vi "fgv_debug.vi"(7 "Operation":enum16{"Reset", "ReadCommand", "SetCommand"}(ring)=enum."ReadCommand", 8 "error in":errorcluster, 9 "Command in":string, 11 "VISA resource name":refnum<visa-resource-name>) -> (0 "error out":errorcluster, 3 "VISA resource name out":refnum<visa-resource-name>)   [LabVIEW 2014, in "rszvl_rsidr_core.lvlib"]
uses:
  rszvl_rsidr_core.lvlib
  type_Error_Codes.ctl
  Match Regular Expression.xnode
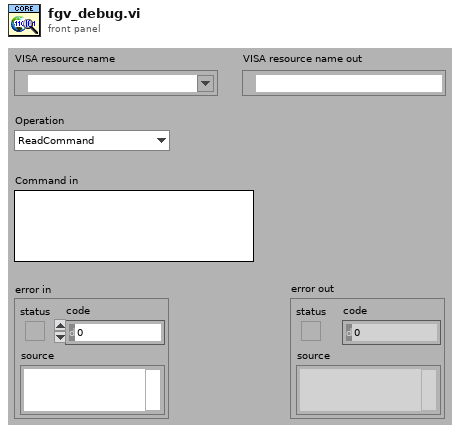
[diagram p1: front panel]
types:
  T1 = typedef "rszvl_rsidr_core.lvlib/type_Error_Codes.ctl" = enum16{"No_error", "VISA_err_ResourceNotFound", "VISA_err_Timeout", "VISA_warn_MoreDataAvailable", "RS_err_MissingCallback", "RS_err_InvalidAttribute", "RS_err_InvalidValue", "RS_err_UnknownResource", "RS_err_AlreadyInitialized", "RS_err_InstrumentStatus", "RS_err_BadRepCapName", "RS_err_TypesMismatch", "RS_err_ValueNotSupported", "RS_err_InvalidRngTable", "RS_err_IDqueryFail", "RS_err_UnexpResponse", "VISA_warn_ConfigNotLoaded", "RS_err_AttributeNotReadable", "RS_err_AttributeNotWritable", "RS_err_InstrumentType", "RS_err_InstrumentOption", "VISA_err_InvalidSize", "RS_err_ReliabilityIndicator", "VISA_warn_UnknownStatus", "VISA_warn_TermCharRead", "VISA_err_IO_error"}
  T2 = typedef "rszvl_rsidr_core.lvlib/type_Session_Data.ctl" = cluster{"Instr type":string, "Instr type for err. msg.":string, "Installed Options":string[], "OPC Timeout":i32, "Query Instrument Status":bool, "Check Range":bool, "Check Options":bool, "Add LF to Write":bool, "Simulate":bool, "Logging":bool, "Logging params":variant, "Interface Type":enum16{"Unknown", "GPIB", "VXI", "GPIB_VXI", "ASRL", "PXI", "TCPIP", "USB", "SOCKET"}, "Fast Sweep":i32, "AdditionalFlags":i32, "WaitBeforeWrite":i32, "WaitBeforeRead":i32, "BinDataChunkSize":i64}
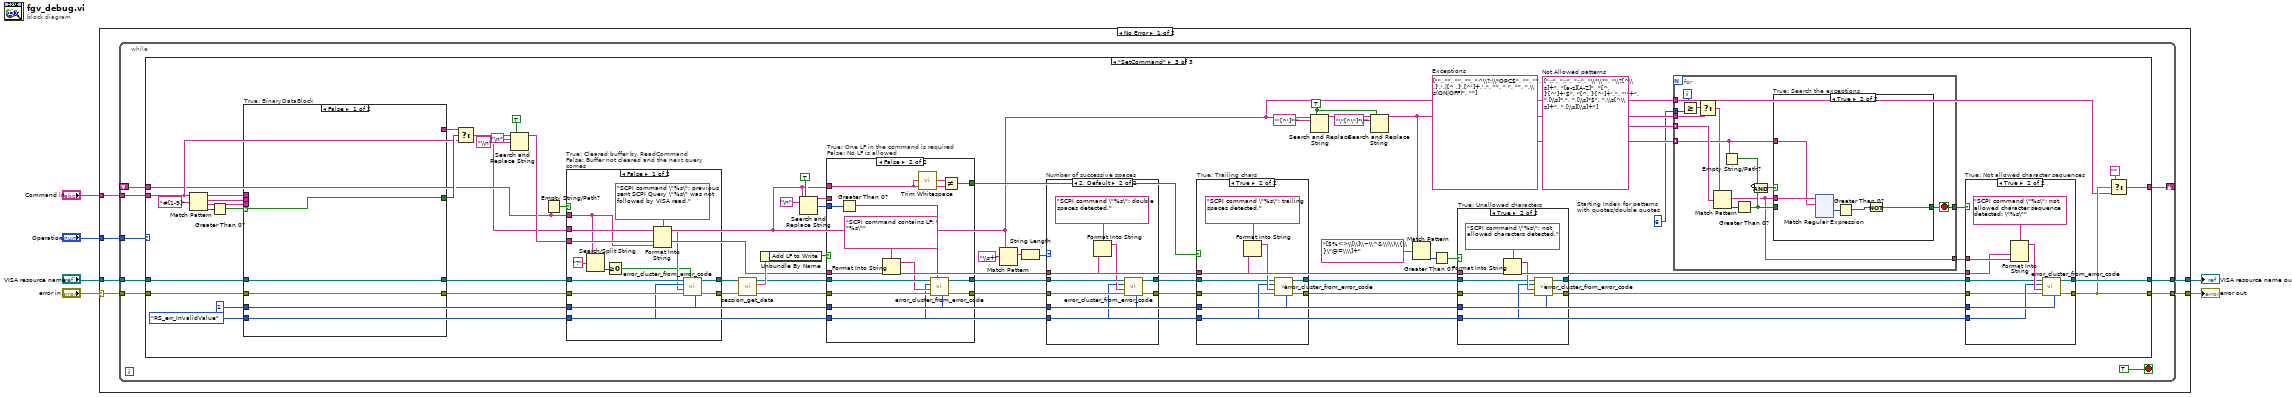
[diagram p0: block diagram]
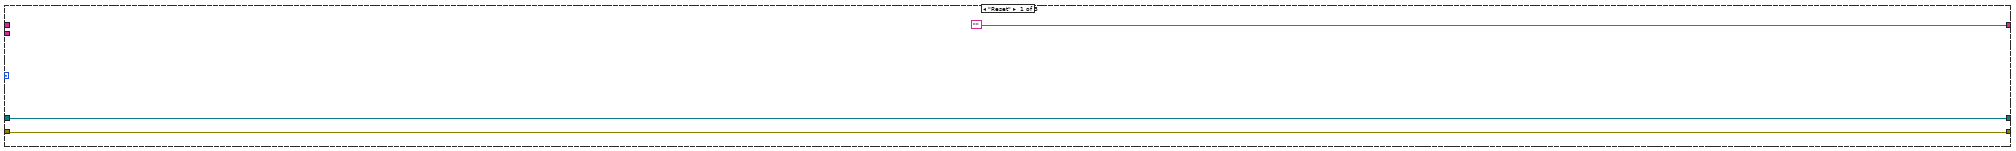
[diagram p2: hidden frame]
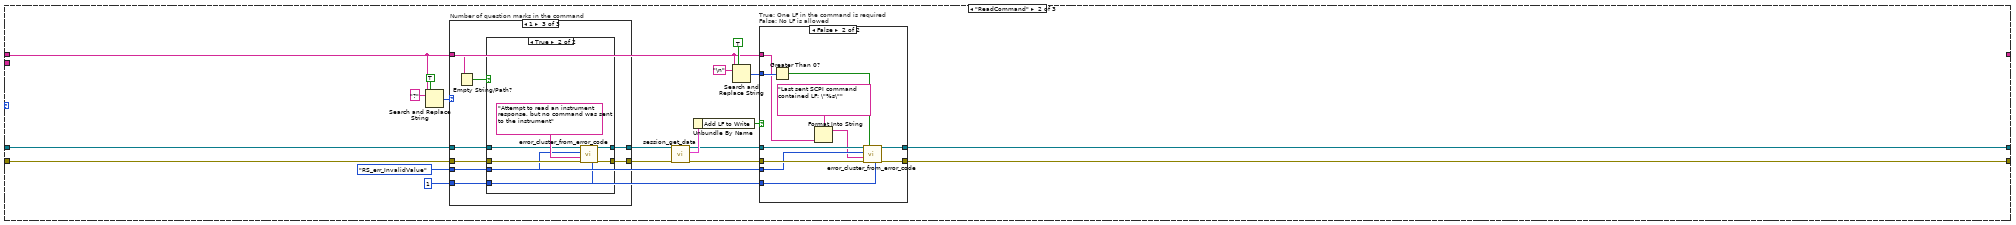
[diagram p3: hidden frame]
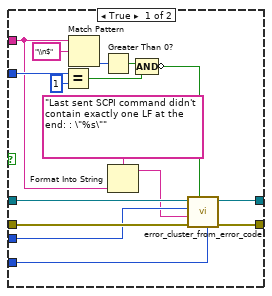
[diagram p4: hidden frame]
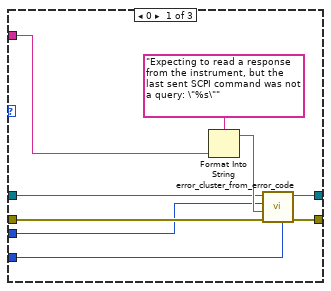
[diagram p5: hidden frame]
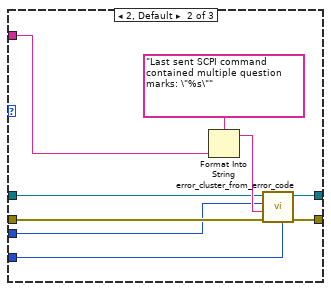
[diagram p6: hidden frame]
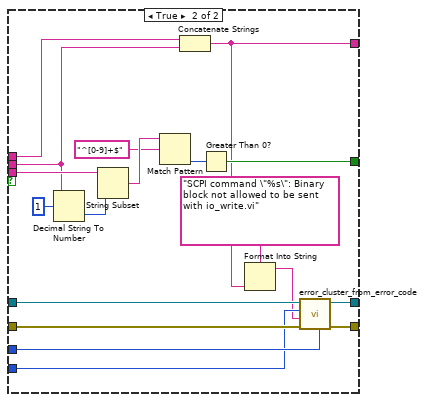
[diagram p8: hidden frame]
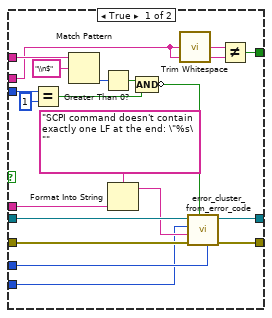
[diagram p13: hidden frame]
diagram:
  n1 = case shown="No Error" "error in" {
    selector: "error in" -> [w8 w414]
    tunnel: [w10 w414] -> w2
    tunnel: "Operation" -> [w12 _]
    tunnel: "Command in" -> [w11 _]
    tunnel: "VISA resource name" -> [w7 w413]
    tunnel: [w9 w413] -> w1
    frame No Error {
      n2 = while {
        shift-right: [w18] -> _
        shift-left: _ -> [w17]
        tunnel: w12 -> [w20]
        tunnel: w8 -> [w14]
        tunnel: w11 -> [w19]
        tunnel: w7 -> [w13]
        tunnel: [w16] -> w10
        tunnel: [w15] -> w9
        stop <- TRUE stop-if-true
        n3 = case shown="\"SetCommand\"" w20 {
          tunnel: w19 -> [_ _ w125]
          tunnel: ["" ("Empty String Constant") _ w161] -> w18
          tunnel: w17 -> [_ w28 w124]
          tunnel: w14 -> [w23 w40 w110]
          tunnel: w13 -> [w22 w39 w109]
          tunnel: [w23 w27 w140] -> w16
          tunnel: [w22 w26 w141] -> w15
          frame "Reset" {
          }
          frame "ReadCommand" {
            w25 = 1 ("Cut first x elements\nfrom Error Chain (0)")
            w31 = type_Error_Codes."RS_err_InvalidValue" ("Error Enum in")
            n4 = Search and Replace String(replace all?=TRUE ("replace all? (F)"), input string=w28, search string="?") -> (number of replacements=w41:i32)  [unwired: 5 in, 3 out]
            n5 = case "Number of question marks in the command" shown="1" w41 {
              tunnel: w40 -> [w78 w87 w94]
              tunnel: [w77 w86 w92] -> w38
              tunnel: w28 -> [w76 w85 w96]
              tunnel: w39 -> [w74 w82 w93]
              tunnel: [w73 w84 w91] -> w37
              tunnel: w31 -> [w72 w81 w90]
              tunnel: w25 -> [w71 w80 w89]
              frame 0 {
                n6 = Format Into String(format string="Expecting to read a response from the instrument, but the last sent SCPI command was not a query: \"%s\"", w76) -> (resulting string=w75:string)  [unwired: 2 in, 1 out]
                n7 = call "error_cluster_from_error_code.vi"("Cut first x elements\nfrom Error Chain (0)"=w71, "error in"=w78, "error message (\"\")"=w75, "Error Enum in"=w72, "VISA resource name"=w74) -> ("error out"=w77:errorcluster, "VISA resource name out"=w73:refnum<visa-resource-name>)  [unwired: 5 in]
              }
              frame 2, Default {
                n8 = Format Into String(format string="Last sent SCPI command contained multiple question marks: \"%s\"", w85) -> (resulting string=w83:string)  [unwired: 2 in, 1 out]
                n9 = call "error_cluster_from_error_code.vi"("Cut first x elements\nfrom Error Chain (0)"=w80, "error in"=w87, "error message (\"\")"=w83, "Error Enum in"=w81, "VISA resource name"=w82) -> ("error out"=w86:errorcluster, "VISA resource name out"=w84:refnum<visa-resource-name>)  [unwired: 5 in]
              }
              frame 1 {
                n10 = Empty String/Path?(string/path=w96) -> (empty?=w95:bool)
                n11 = case shown="True" w95 {
                  tunnel: w94 -> [w98 w104]
                  tunnel: [w98 w102] -> w92
                  tunnel: w93 -> [w97 w103]
                  tunnel: [w97 w101] -> w91
                  tunnel: w90 -> [_ w100]
                  tunnel: w89 -> [_ w99]
                  frame False {
                  }
                  frame True {
                    n12 = call "error_cluster_from_error_code.vi"("Cut first x elements\nfrom Error Chain (0)"=w99, "error in"=w104, "error message (\"\")"="Attempt to read an instrument response, but no command was sent to the instrument" ("error message (\"\")"), "Error Enum in"=w100, "VISA resource name"=w103) -> ("error out"=w102:errorcluster, "VISA resource name out"=w101:refnum<visa-resource-name>)  [unwired: 5 in]
                  }
                }
              }
            }
            n13 = call "session_get_data.vi"("error in"=w38, "VISA resource name"=w37) -> ("error out"=w33:errorcluster, "Session User Data out"=w34:T2, "VISA resource name out"=w32:refnum<visa-resource-name>)  [unwired: 7 in]
            n14 = Unbundle By Name(w34) -> ("Add LF to Write"=w30:bool)
            n15 = Search and Replace String(replace all?=TRUE ("replace all? (F)"), input string=w28, search string="\n" ("Line Feed Constant")) -> (number of replacements=w29:i32)  [unwired: 5 in, 3 out]
            n16 = case "True: One LF in the command is required\nFalse: No LF is allowed" shown="False" w30 {
              tunnel: w33 -> [w59 w70]
              tunnel: w32 -> [w58 w69]
              tunnel: w31 -> [w57 w68]
              tunnel: w29 -> [w56 w65]
              tunnel: w28 -> [w46 w61]
              tunnel: [w49 w67] -> w27
              tunnel: [w48 w66] -> w26
              tunnel: w25 -> [w44 w60]
              frame True {
                n17 = Equal?(x=w56, y=1) -> (x = y?=w51:bool)
                n18 = Match Pattern(string=w46, regular expression="\\n$") -> (offset past match=w53:i32)  [unwired: 1 in, 3 out]
                n19 = Greater Than 0?(x=w53) -> (x > 0?=w52:bool)
                n20 = Format Into String(format string="Last sent SCPI command didn't contain exactly one LF at the end: : \"%s\"", w46) -> (resulting string=w45:string)  [unwired: 2 in, 1 out]
                n21 = Compound Arithmetic op=AND(w52, w51) -> (invert w50:bool)
                n22 = call "error_cluster_from_error_code.vi"("Cut first x elements\nfrom Error Chain (0)"=w44, "error creation enabled (T)"=w50, "error in"=w59, "error message (\"\")"=w45, "Error Enum in"=w57, "VISA resource name"=w58) -> ("error out"=w49:errorcluster, "VISA resource name out"=w48:refnum<visa-resource-name>)  [unwired: 4 in]
              }
              frame False {
                n23 = Greater Than 0?(x=w65) -> (x > 0?=w64:bool)
                n24 = Format Into String(format string="Last sent SCPI command contained LF: \"%s\"", w61) -> (resulting string=w62:string)  [unwired: 2 in, 1 out]
                n25 = call "error_cluster_from_error_code.vi"("Cut first x elements\nfrom Error Chain (0)"=w60, "error creation enabled (T)"=w64, "error in"=w70, "error message (\"\")"=w62, "Error Enum in"=w68, "VISA resource name"=w69) -> ("error out"=w67:errorcluster, "VISA resource name out"=w66:refnum<visa-resource-name>)  [unwired: 4 in]
              }
            }
          }
          frame "SetCommand" {
            w116 = 6  # Starting Index for patterns with quotes/double quotes
            w130 = string[] ["", "", "", "", "^\\?;\\*OPC$", "", "", "[^ ,]','.|[^ ,]',[^']+,'.", "", " ", "", ",\\s(ON|OFF)", ""]  # Exceptions
            w121 = TRUE ("replace all? (F)")
            w145 = string[] ["::", ";;", ":;", "\\*\\*", "\\?[^\\s]+", "[a-z][A-Z]", "[^, ]'[^']+'$", "[^, ]'[^']+'.", "''+", ",[\\s]*,", ",[\\s]*$", ",\\s[^\\s]+", ",[\\s][\\s]+"]  # Not Allowed patterns
            w111 = 1 ("Cut first x elements\nfrom Error Chain (0)")
            w106 = type_Error_Codes."RS_err_InvalidValue" ("Error Enum in")
            n26 = Match Pattern(string=w125, regular expression="#[1-9]") -> (before substring=w113:string, match substring=w115:string, after substring=w127:string, offset past match=w129:i32)  [unwired: 1 in]
            n27 = Greater Than 0?(x=w129) -> (x > 0?=w128:bool)
            n28 = case "True: BinaryDataBlock" shown="False" w128 {
              selector: w128 -> [w169 _]
              tunnel: w127 -> [_ w186]
              tunnel: w115 -> [_ w179]
              tunnel: [w169 w181] -> w126
              tunnel: [_ w170] -> w114
              tunnel: w113 -> [_ w180]
              tunnel: w111 -> [_ w174]
              tunnel: w110 -> [w167 w178]
              tunnel: w109 -> [w168 w177]
              tunnel: [w167 w176] -> w108
              tunnel: [w168 w175] -> w107
              tunnel: w106 -> [_ w173]
              frame False {
              }
              frame True {
                n29 = Decimal String To Number(string=w179, offset=1) -> (number=w185:i32)  [unwired: 1 in, 1 out]
                n30 = String Subset(string=w186, length (rest)=w185) -> (substring=w184:string)  [unwired: 1 in]
                n31 = Match Pattern(string=w184, regular expression="^[0-9]+$") -> (offset past match=w182:i32)  [unwired: 1 in, 3 out]
                n32 = Concatenate Strings(w180, w179) -> (w170:string)
                n33 = Greater Than 0?(x=w182) -> (x > 0?=w181:bool)
                n34 = Format Into String(format string="SCPI command \"%s\": Binary block not allowed to be sent with io_write.vi", w170) -> (resulting string=w171:string)  [unwired: 2 in, 1 out]
                n35 = call "error_cluster_from_error_code.vi"("Cut first x elements\nfrom Error Chain (0)"=w174, "error in"=w178, "error message (\"\")"=w171, "Error Enum in"=w173, "VISA resource name"=w177) -> ("error out"=w176:errorcluster, "VISA resource name out"=w175:refnum<visa-resource-name>)  [unwired: 5 in]
              }
            }
            n36 = Select(t=w114, s=w126, f=w125) -> (s? t:f=w117:string)
            n37 = Search and Replace String(replace all?=TRUE ("replace all? (F)"), input string=w117, search string="\n" ("Line Feed Constant"), replace string="\\n" ("input string")) -> (result string=w132:string)  [unwired: 4 in, 3 out]
            n38 = Empty String/Path?(string/path=w124) -> (empty?=w162:bool)
            n39 = case "True: Cleared buffer by ReadCommand\nFalse: Buffer not cleared and the next query comes" shown="False" w162 {
              tunnel: w124 -> [w405 _]
              tunnel: w108 -> [w409 w412]
              tunnel: [w408 w412] -> w152
              tunnel: w117 -> [_ _]
              tunnel: w111 -> [w404 _]
              tunnel: w106 -> [w403 _]
              tunnel: w107 -> [w402 w411]
              tunnel: [w401 w411] -> w153
              tunnel: w132 -> [w398 _]
              frame False {
                n40 = Search/Split String(string=w405, search string/char (-)="?") -> (offset of match=w407:i32)  [unwired: 1 in, 2 out]
                n41 = Greater Or Equal To 0?(x=w407) -> (x >= 0?=w399:bool)
                n42 = Format Into String(format string="SCPI command \"%s\": previous sent SCPI Query \"%s\" was not followed by VISA read.", w398, w405) -> (resulting string=w400:string)  [unwired: 2 in, 1 out]
                n43 = call "error_cluster_from_error_code.vi"("Cut first x elements\nfrom Error Chain (0)"=w404, "error creation enabled (T)"=w399, "error in"=w409, "error message (\"\")"=w400, "Error Enum in"=w403, "VISA resource name"=w402) -> ("error out"=w408:errorcluster, "VISA resource name out"=w401:refnum<visa-resource-name>)  [unwired: 4 in]
              }
              frame True {
              }
            }
            n44 = call "session_get_data.vi"("error in"=w152, "VISA resource name"=w153) -> ("error out"=w157:errorcluster, "Session User Data out"=w158:T2, "VISA resource name out"=w156:refnum<visa-resource-name>)  [unwired: 7 in]
            n45 = Unbundle By Name(w158) -> ("Add LF to Write"=w155:bool)
            n46 = Search and Replace String(replace all?=TRUE ("replace all? (F)"), input string=w117, search string="\n" ("Line Feed Constant")) -> (result string=w119:string, number of replacements=w154:i32)  [unwired: 5 in, 2 out]
            n47 = case "True: One LF in the command is required\nFalse: No LF is allowed" shown="False" w155 {
              tunnel: w157 -> [w372 w386]
              tunnel: w156 -> [w371 w385]
              tunnel: w154 -> [w370 w382]
              tunnel: w117 -> [w360 w374]
              tunnel: [w363 w384] -> w150
              tunnel: [w362 w383] -> w151
              tunnel: w111 -> [w358 w378]
              tunnel: w106 -> [w357 w377]
              tunnel: w132 -> [w356 w376]
              tunnel: w119 -> [w354 _]
              tunnel: [w353 w373] -> w118
              frame True {
                n48 = Equal?(x=w370, y=1) -> (x = y?=w365:bool)
                n49 = Match Pattern(string=w360, regular expression="\\n$") -> (offset past match=w367:i32)  [unwired: 1 in, 3 out]
                n50 = Greater Than 0?(x=w367) -> (x > 0?=w366:bool)
                n51 = Format Into String(format string="SCPI command doesn't contain exactly one LF at the end: \"%s\"", w356) -> (resulting string=w359:string)  [unwired: 2 in, 1 out]
                n52 = Compound Arithmetic op=AND(w366, w365) -> (invert w364:bool)
                n53 = call "Trim Whitespace.vi"("string"=w354) -> ("trimmed string"=w355:string)  [unwired: 1 in]
                n54 = call "error_cluster_from_error_code.vi"("Cut first x elements\nfrom Error Chain (0)"=w358, "error creation enabled (T)"=w364, "error in"=w372, "error message (\"\")"=w359, "Error Enum in"=w357, "VISA resource name"=w371) -> ("error out"=w363:errorcluster, "VISA resource name out"=w362:refnum<visa-resource-name>)  [unwired: 4 in]
                n55 = Not Equal?(x=w355, y=w354) -> (x != y?=w353:bool)
              }
              frame False {
                n56 = Greater Than 0?(x=w382) -> (x > 0?=w381:bool)
                n57 = Format Into String(format string="SCPI command contains LF: \"%s\"", w376) -> (resulting string=w379:string)  [unwired: 2 in, 1 out]
                n58 = call "Trim Whitespace.vi"("string"=w374) -> ("trimmed string"=w375:string)  [unwired: 1 in]
                n59 = call "error_cluster_from_error_code.vi"("Cut first x elements\nfrom Error Chain (0)"=w378, "error creation enabled (T)"=w381, "error in"=w386, "error message (\"\")"=w379, "Error Enum in"=w377, "VISA resource name"=w385) -> ("error out"=w384:errorcluster, "VISA resource name out"=w383:refnum<visa-resource-name>)  [unwired: 4 in]
                n60 = Not Equal?(x=w375, y=w374) -> (x != y?=w373:bool)
              }
            }
            n61 = Match Pattern(string=w117, regular expression="\\s+") -> (match substring=w165:string)  [unwired: 1 in, 3 out]
            n62 = String Length(string=w165) -> (length=w166:i32)
            n63 = case "Number of successive spaces" shown="2, Default" w166 {
              tunnel: w150 -> [w388 w397]
              tunnel: [w388 w396] -> w139
              tunnel: w151 -> [w387 w394]
              tunnel: [w387 w393] -> w138
              tunnel: w111 -> [_ w391]
              tunnel: w106 -> [_ w390]
              tunnel: w132 -> [_ w389]
              frame 0, 1 {
              }
              frame 2, Default {
                n64 = Format Into String(format string="SCPI command \"%s\": double spaces detected.", w389) -> (resulting string=w392:string)  [unwired: 2 in, 1 out]
                n65 = call "error_cluster_from_error_code.vi"("Cut first x elements\nfrom Error Chain (0)"=w391, "error in"=w397, "error message (\"\")"=w392, "Error Enum in"=w390, "VISA resource name"=w394) -> ("error out"=w396:errorcluster, "VISA resource name out"=w393:refnum<visa-resource-name>)  [unwired: 5 in]
              }
            }
            n66 = case "True: Trailing chars" shown="True" w118 {
              tunnel: w139 -> [w189 w194]
              tunnel: [w189 w192] -> w137
              tunnel: w138 -> [w188 w193]
              tunnel: [w188 w191] -> w136
              tunnel: w111 -> [_ w196]
              tunnel: w106 -> [_ w195]
              tunnel: w132 -> [_ w190]
              frame False {
              }
              frame True {
                n67 = Format Into String(format string="SCPI command \"%s\": trailing spaces detected.", w190) -> (resulting string=w197:string)  [unwired: 2 in, 1 out]
                n68 = call "error_cluster_from_error_code.vi"("Cut first x elements\nfrom Error Chain (0)"=w196, "error in"=w194, "error message (\"\")"=w197, "Error Enum in"=w195, "VISA resource name"=w193) -> ("error out"=w192:errorcluster, "VISA resource name out"=w191:refnum<visa-resource-name>)  [unwired: 5 in]
              }
            }
            n69 = Search and Replace String(replace all?=w121, input string=w117, search string="'[^']*'" ("regular expression")) -> (result string=w122:string)  [unwired: 5 in, 3 out]
            n70 = Search and Replace String(replace all?=w121, input string=w122, search string="\"[^\"]*\"" ("regular expression")) -> (result string=w123:string)  [unwired: 5 in, 3 out]
            n71 = Match Pattern(string=w123, regular expression="[$%<>\\[\\]\\~\\^&\\(\\)\\{\\}\"@=\\\\]+") -> (offset past match=w147:i32)  [unwired: 1 in, 3 out]
            n72 = Greater Than 0?(x=w147) -> (x > 0?=w148:bool)
            n73 = case "True: Unallowed characters" shown="True" w148 {
              tunnel: w137 -> [w343 w348]
              tunnel: [w343 w346] -> w142
              tunnel: w136 -> [w342 w347]
              tunnel: [w342 w345] -> w146
              tunnel: w111 -> [_ w350]
              tunnel: w106 -> [_ w349]
              tunnel: w132 -> [_ w344]
              frame False {
              }
              frame True {
                n74 = Format Into String(format string="SCPI command \"%s\": not allowed characters detected.", w344) -> (resulting string=w351:string)  [unwired: 2 in, 1 out]
                n75 = call "error_cluster_from_error_code.vi"("Cut first x elements\nfrom Error Chain (0)"=w350, "error in"=w348, "error message (\"\")"=w351, "Error Enum in"=w349, "VISA resource name"=w347) -> ("error out"=w346:errorcluster, "VISA resource name out"=w345:refnum<visa-resource-name>)  [unwired: 5 in]
              }
            }
            n76 = for {
              tunnel: w145 -> [w212] mode=indexing
              tunnel: [w205] -> w144
              tunnel: [w207] -> w143
              tunnel: w123 -> [w201]
              tunnel: w130 -> [w206] mode=indexing
              tunnel: w117 -> [w204]
              tunnel: w116 -> [w200]
              i -> [w203]
              stop <- w205 stop-if-true
              n77 = Greater Or Equal?(x=w203, y=w200) -> (x >= y?=w202:bool)
              n78 = Select(t=w204, s=w202, f=w201) -> (s? t:f=w199:string)
              n79 = Match Pattern(string=w199, regular expression=w212) -> (match substring=w207:string, offset past match=w211:i32)  [unwired: 1 in, 2 out]
              n80 = Empty String/Path?(string/path=w206) -> (empty?=w210:bool)
              n81 = Greater Than 0?(x=w211) -> (x > 0?=w208:bool)
              n82 = Compound Arithmetic op=AND(invert w210, w208) -> (w209:bool)
              n83 = case "True: Search the exceptions" shown="True" w209 {
                tunnel: w208 -> [w213 _]
                tunnel: w207 -> [_ w217]
                tunnel: w206 -> [_ w214]
                tunnel: [w213 w218] -> w205
                frame False {
                }
                frame True {
                  n84 = xnode ("Match Regular Expression")("input string"=w217, "regular expression"=w214) -> ("offset past match"=w216:i32)  [unwired: 4 in, 4 out]
                  n85 = Greater Than 0?(x=w216) -> (x > 0?=w215:bool)
                  n86 = Not(x=w215) -> (.not. x?=w218:bool)
                }
              }
            }
            n87 = case "True: Not allowed character sequences" shown="True" w144 {
              tunnel: w142 -> [w331 w337]
              tunnel: [w331 w335] -> w140
              tunnel: w146 -> [w330 w336]
              tunnel: [w330 w334] -> w141
              tunnel: w111 -> [_ w339]
              tunnel: w106 -> [_ w338]
              tunnel: w143 -> [_ w333]
              tunnel: w132 -> [_ w332]
              frame False {
              }
              frame True {
                n88 = Format Into String(format string="SCPI command \"%s\": not allowed character sequence detected: \"%s\"", w332, w333) -> (resulting string=w340:string)  [unwired: 2 in, 1 out]
                n89 = call "error_cluster_from_error_code.vi"("Cut first x elements\nfrom Error Chain (0)"=w339, "error in"=w337, "error message (\"\")"=w340, "Error Enum in"=w338, "VISA resource name"=w336) -> ("error out"=w335:errorcluster, "VISA resource name out"=w334:refnum<visa-resource-name>)  [unwired: 5 in]
              }
            }
            n90 = Select(t="" ("Empty String Constant"), s=w140, f=w117) -> (s? t:f=w161:string)
          }
        }
      }
    }
    frame Error {
    }
  }
  "error out" <- w2
  "VISA resource name out" <- w1
